vi "LabViewV1.4.0.vi"() -> ()   [LabVIEW 2020]
uses:
  <vilib>/DAQmx/read.llb/DAQmx Read (Analog 2D DBL NChan NSamp).vi
  <vilib>/Analysis/baseanly.llb/Mean (DBL).vi
  <vilib>/DAQmx/miscellaneous.llb/DAQmx Fill In Error Info.vi
  <vilib>/Analysis/NI_AALBase.lvlib
  <resource>/objmgr/daqmx.rc
panel:
  out "Numeric 2":i32
  out "Numeric":i32
  out "index of Module 3":i32
  out "index of Module 2":i32
  out "double precision float":dbl
  out "Time Stamp":timestamp=timestamp(-21600 s since 1904-01-01)
  out "subarray 2":string[](array[string])
  out "index of Module 1":i32
  out "subarray":string[](array[string])
  in  "Counter":dbl
  out ".not. (x .or. y)?":bool
  out "index of element":i32
  out "element":dbl
  out "?":timestamp
  out "Channels":refnum<k21>[](array[refnum])
  out "size(s)":i32
  out "NumDevices":u32
  out "x/y":dbl
  in  "?":T1(tab)
  out "Sampling Status":bool
  in  "Sampling Time":u32=5
  in  "Read Time (s)":u32=60
  in  "Channel List":string(combo)="Temperature"
  out "Read Count Daily":string="0" caption="Timestamp"
  out "Countdown to Read":string="0\n 6:17:48 PM" caption="Timestamp"
  out "?":string="Timestamp"
  out "?":string="File Location"
  out "Timestamp":string="7/26/2020\n 6:17:48 PM"
  in  "Start":bool
  in  "Next Button":bool
  in  "Stop Button 2":bool
  out "Graph Running":bool
  in  "Resolution":u8=10 min=10
  in  "Stop Button":bool
  in  "Play Button":bool
  out "Module 3":bool
  out "Module 2":bool
  out "Module 1":bool
  out "3":bool
  out "2":bool
  out "1":bool
  in  "Running Module":u8=1 min=1 max=3
  in  "Module 3 Task":refnum<k21>="MyTemperatureTask_2"
  out "?":waveform(dbl)(graph)
  in  "Module 3 File Data Location":path=path "E:/KMUTT/Master Degree/labviewjgsee/log/Module3"
  in  "Module 2 File Data Location":path=path "E:/KMUTT/Master Degree/labviewjgsee/log/Module2"
  in  "Module 2 Task":refnum<k21>="MyTemperatureTask_1"
  in  "Module 1 File Data Location":path=path "E:/KMUTT/Master Degree/labviewjgsee/log/Module1"
  in  "Module 1 Task":refnum<k21>="MyTemperatureTask"
  in  "DAQmx Device Name":tag="JGSEE"
  out "Tnp_in":dbl format="%#_4g"
  out "T_head":dbl format="%#_4g"
  out "Tnw":dbl format="%#_4g"
  out "Trp_out":dbl format="%#_4g"
  out "Trp_in":dbl format="%#_4g"
  out "Tww_o":dbl format="%#_4g"
  out "Tew_o":dbl format="%#_4g"
  out "Tsw_o":dbl format="%#_4g"
  out "Tnw_o":dbl format="%#_4g"
  out "3_inlet_HE":dbl format="%#_4g"
  out "tnp_out":dbl format="%#_4g"
  out "4_outlet_HE":dbl format="%#_4g"
  out "Tp5":dbl format="%#_4g"
  out "Tp4":dbl format="%#_4g"
  out "Tp3":dbl format="%#_4g"
  out "Tp2":dbl format="%#_4g"
  out "Tp1":dbl format="%#_4g"
  out "Tnp_o":dbl format="%#_4g"
  out "Tfoot":dbl format="%#_4g"
  out "Ttest":dbl format="%#_4g"
  out "T_body":dbl format="%#_4g"
  out "Tshaft_supply":dbl format="%#_4g"
  out "Tshaft_return":dbl format="%#_4g"
  out "Tat":dbl format="%#_4g"
  out "Ta":dbl format="%#_4g"
  out "Tc":dbl format="%#_4g"
  out "Tf":dbl format="%#_4g"
  out "Tsg":dbl format="%#_4g"
  out "Tew":dbl format="%#_4g"
  out "Tng":dbl format="%#_4g"
  out "Tww":dbl format="%#_4g"
  out "Tsw":dbl format="%#_4g"
  out "Table Module 1":string[][](table)
  out "Table Module 2":string[][](table)
  out "Table Module 3":string[][](table)
  in  "Select Channel Module 1":string(combo)
  out "?":string="Date"
  out "Timestamp 2":string="7/26/2020\n 6:17:48 PM" caption="Timestamp"
  out "Graph Module 1":cluster{timestamp[], dbl[]}[](graph)
  in  "Select Channel Module 2":string(combo)
  out "?":string="Date"
  out "Timestamp 3":string="7/26/2020\n 6:17:48 PM" caption="Timestamp"
  out "Graph Module 2":cluster{timestamp[], dbl[]}[](graph)
  in  "Select Channel Module 3":string(combo)
  out "?":string="Date"
  out "Timestamp 4":string="7/26/2020\n 6:17:48 PM" caption="Timestamp"
  out "Graph Module 3":cluster{timestamp[], dbl[]}[](graph)
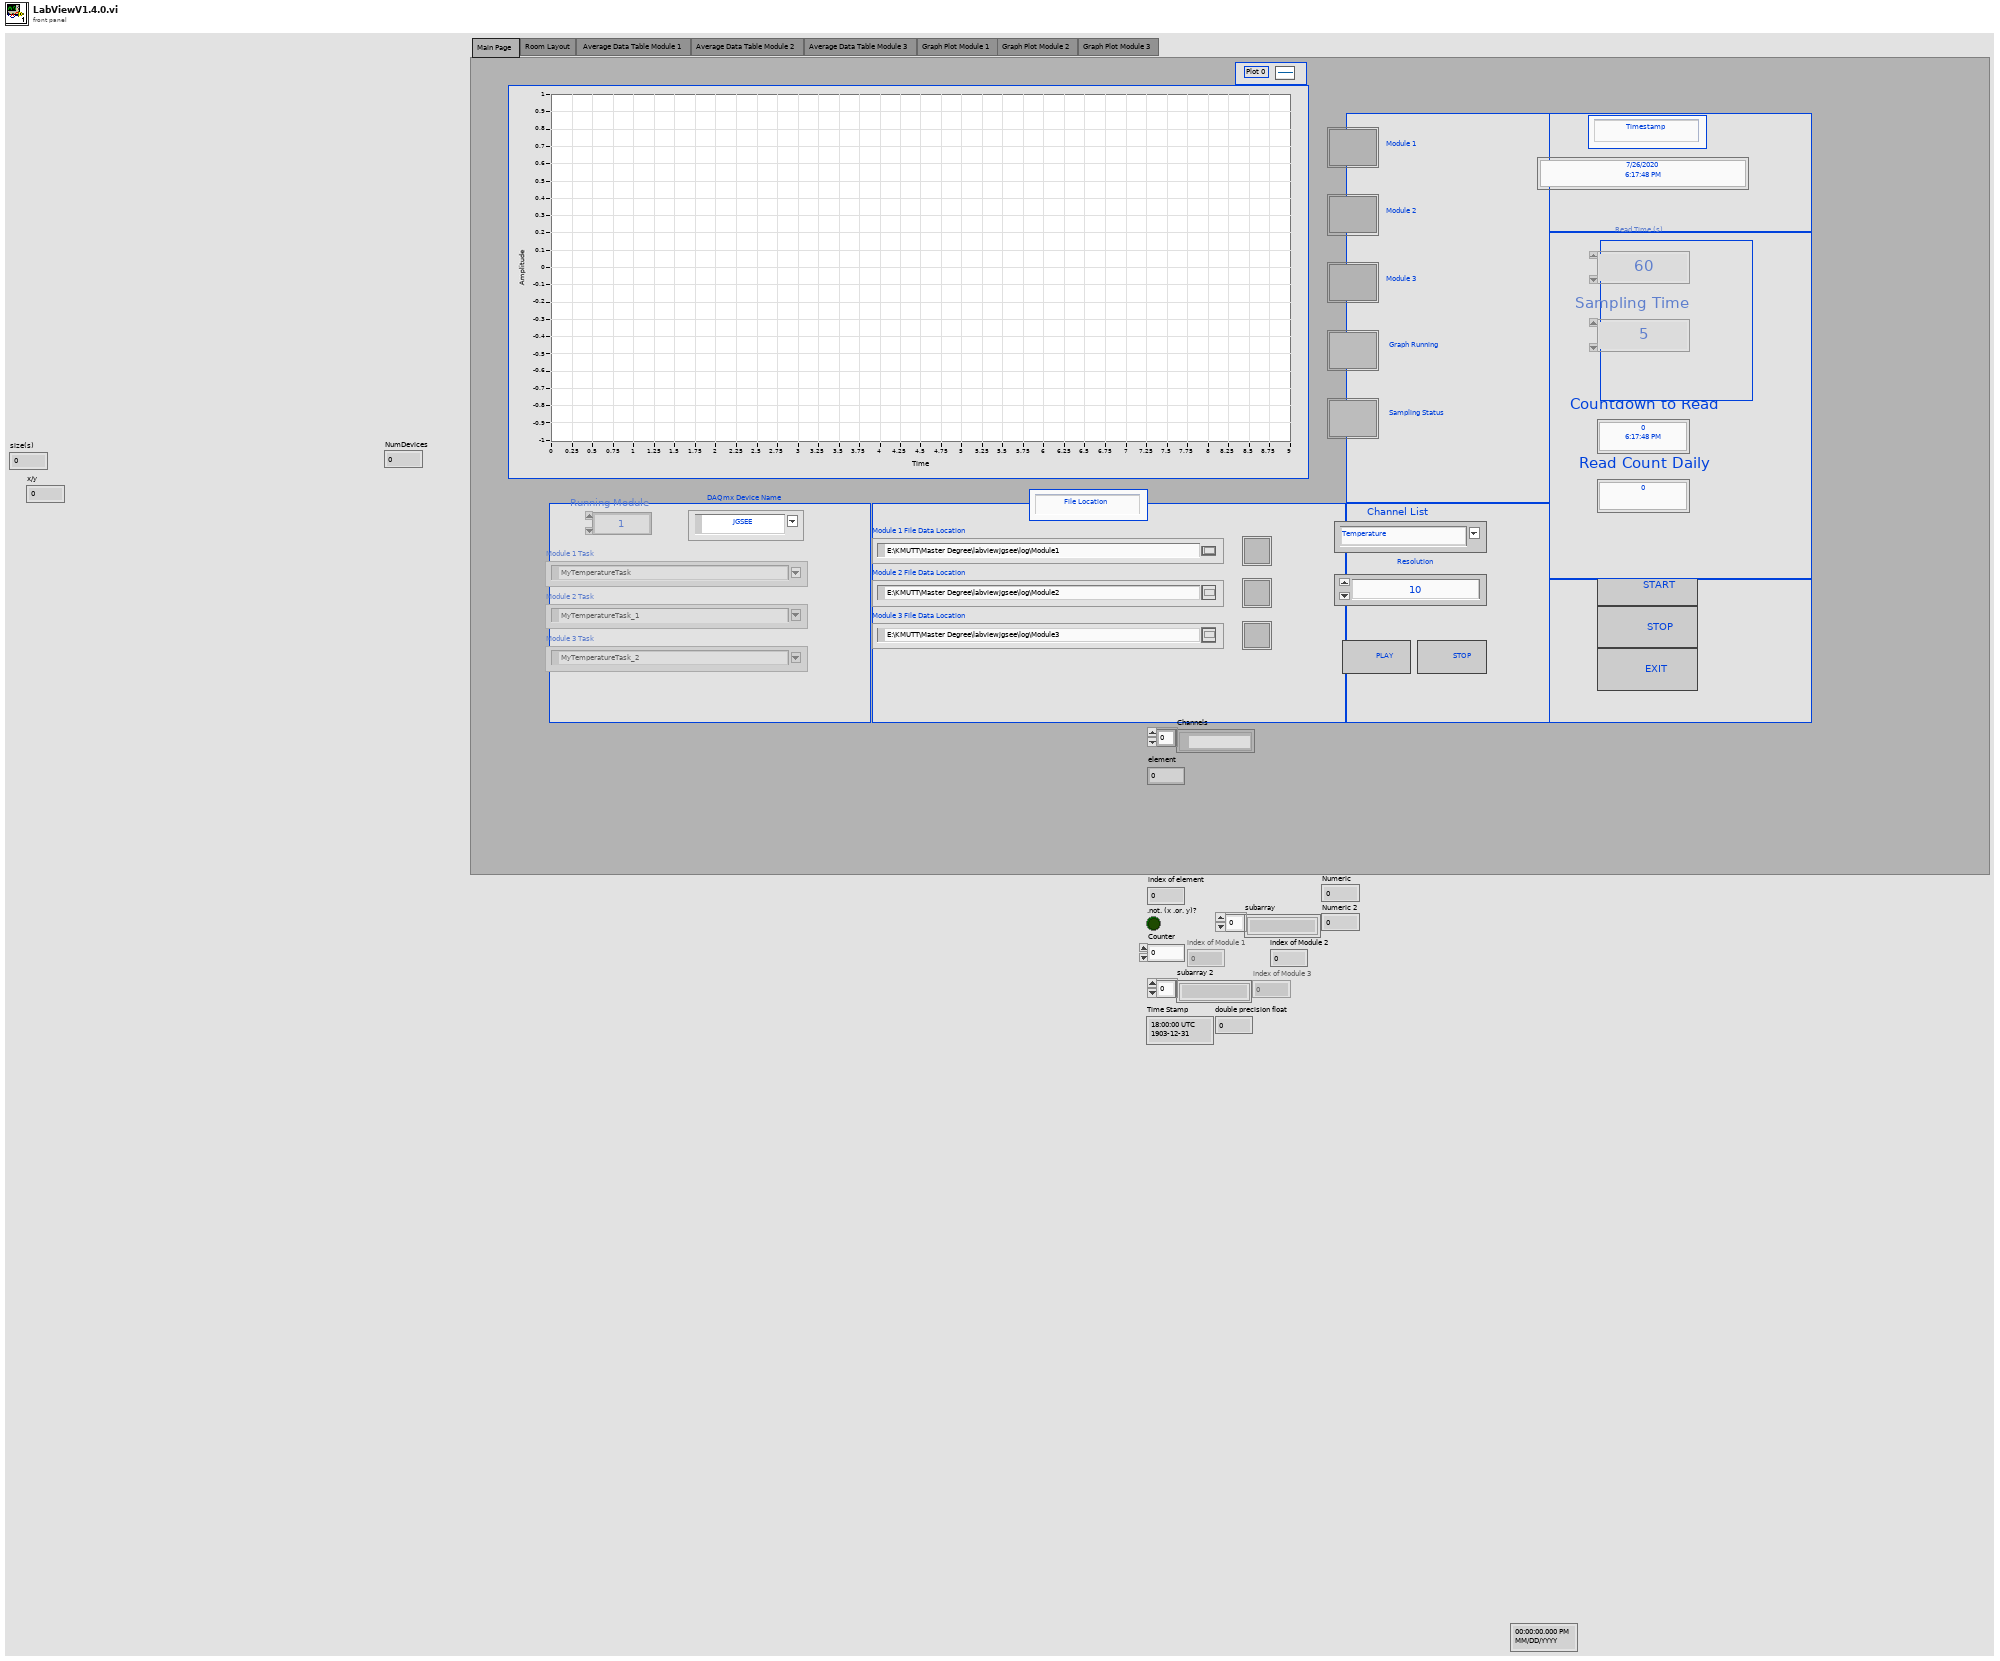
[diagram p1: front panel]
types:
  T1 = enum32{"Main Page ", "Room Layout", " Average Data Table Module 1", "Average Data Table Module 2", "Average Data Table Module 3", "Graph Plot Module 1", "Graph Plot Module 2", "Graph Plot Module 3"}
  T2 = enum16{"open", "replace", "create", "open or create", "replace or create", "replace or create with confirmation"}
  T3 = enum8{"Enabled", "Disabled", "Disabled and Grayed Out"}
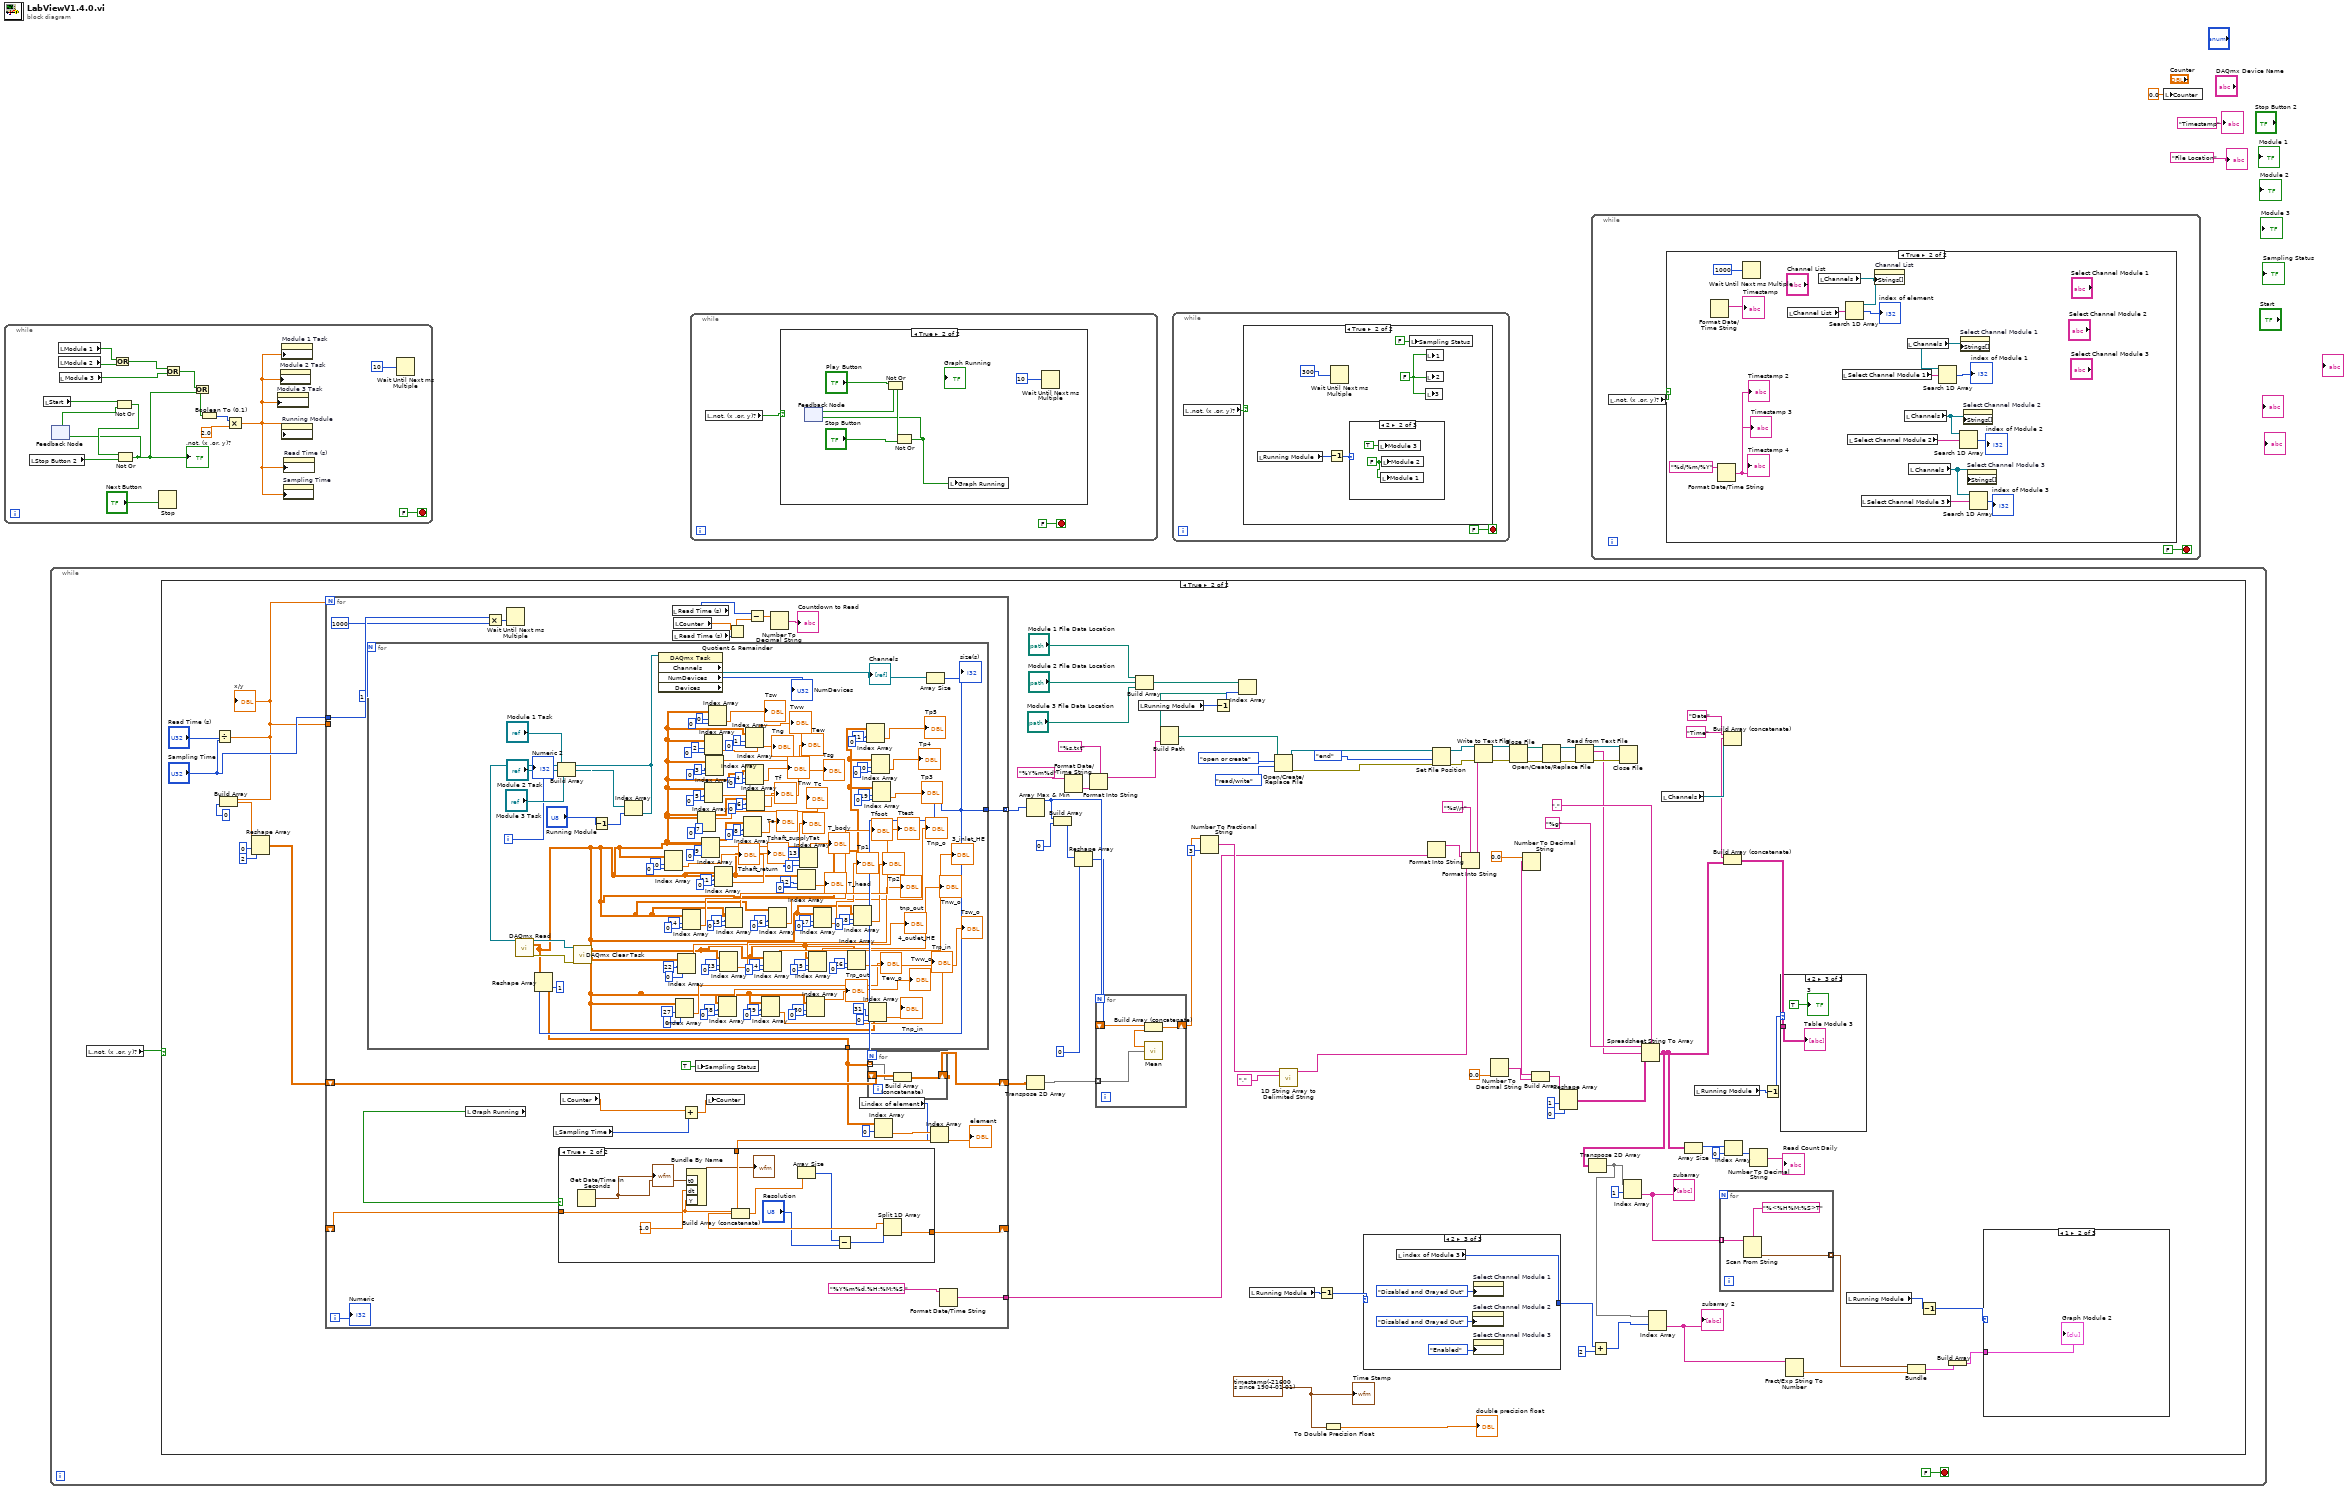
[diagram p0: block diagram]
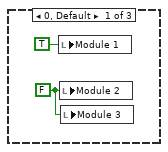
[diagram p4: hidden frame]
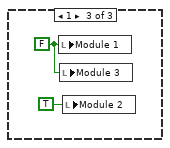
[diagram p5: hidden frame]
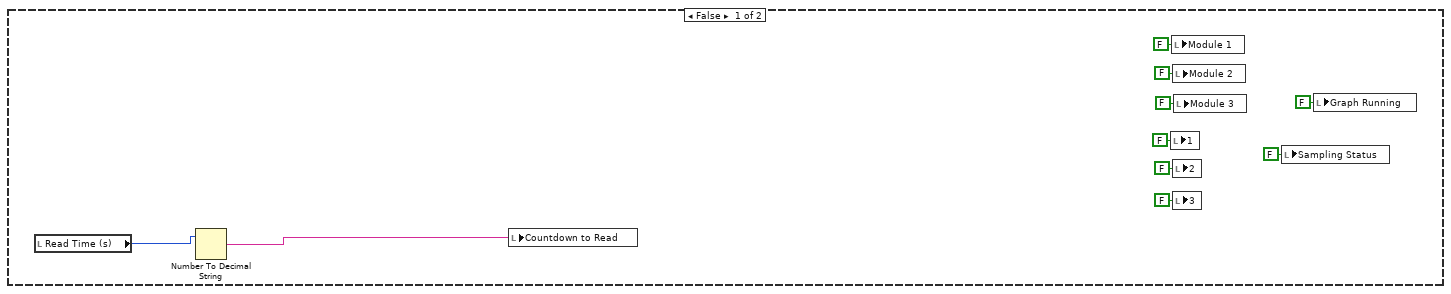
[diagram p7: hidden frame]
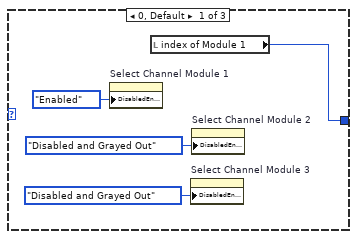
[diagram p8: hidden frame]
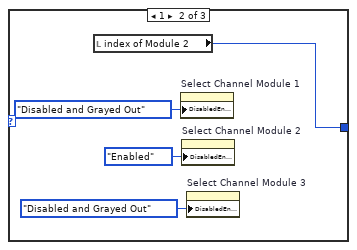
[diagram p9: hidden frame]
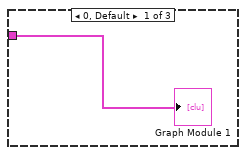
[diagram p10: hidden frame]
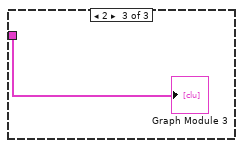
[diagram p11: hidden frame]
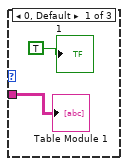
[diagram p12: hidden frame]
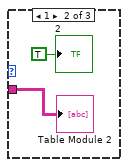
[diagram p13: hidden frame]
diagram:
  n1 = while {
    stop <- FALSE stop-if-true
    n2 = local read "Stop Button 2"() -> (w19:bool)
    n3 = local read "Start"() -> (w15:bool)
    n4 = feedback #1() -> (w17:bool)  [unwired: 1 in]
    n5 = local read "Module 1"() -> (w13:bool)
    n6 = local read "Module 2"() -> (w12:bool)
    n7 = local read "Module 3"() -> (w10:bool)
    n8 = Or(x=w13, y=w12) -> (x .or. y?=w11:bool)
    n9 = Not Or(1:w17, 2:w15) -> (0:w18:bool)
    n10 = Not Or(1:w19, 2:w18) -> (0:w7:bool)
    ".not. (x .or. y)?" <- w7
    n11 = feedback-in #1(w7) -> ()
    n12 = Stop(stop? (T)="Next Button") -> ()
    n13 = Or(x=w11, y=w10) -> (x .or. y?=w9:bool)
    n14 = Or(x=w9, y=w7) -> (x .or. y?=w6:bool)
    n15 = Boolean To (0,1)(Boolean=w6) -> (0, 1=w8:i16)
    n16 = Multiply(x=w8, y=2.0) -> (x*y=w5:dbl)
    n17 = property on="Module 3 Task" class="DAQmxName (strict)"("DisabledEnum"=w5) -> ()  [unwired: 2 in, 2 out]
    n18 = property on="Module 2 Task" class="DAQmxName (strict)"("DisabledEnum"=w5) -> ()  [unwired: 2 in, 2 out]
    n19 = property on="Module 1 Task" class="DAQmxName (strict)"("DisabledEnum"=w5) -> ()  [unwired: 2 in, 2 out]
    n20 = property on="Running Module" class="DigNum (strict)"("DisabledEnum"=w5) -> ()  [unwired: 2 in, 2 out]
    n21 = property on="Sampling Time" class="DigNum (strict)"("DisabledEnum"=w5) -> ()  [unwired: 2 in, 2 out]
    n22 = property on="Read Time (s)" class="DigNum (strict)"("DisabledEnum"=w5) -> ()  [unwired: 2 in, 2 out]
    n23 = Wait Until Next ms Multiple(millisecond multiple=u32 10 ("milliseconds to wait")) -> ()  [unwired: 1 out]
  }
  n24 = while {
    stop <- FALSE stop-if-true
    n25 = local read ".not. (x .or. y)?"() -> (w21:bool)
    n26 = case shown="True" w21 {
      frame False {
        n27 = local read "Read Time (s)"() -> (w24:u32)
        n28 = Number To Decimal String(number=w24) -> (decimal integer string=w23:string)  [unwired: 1 in]
        n29 = local write "Countdown to Read"(w23) -> ()
        n30 = local write "1"(FALSE ("1")) -> ()
        n31 = local write "Module 1"(FALSE ("Module 1")) -> ()
        n32 = local write "Module 2"(FALSE ("Module 2")) -> ()
        n33 = local write "2"(FALSE ("2")) -> ()
        n34 = local write "3"(FALSE ("3")) -> ()
        n35 = local write "Module 3"(FALSE ("Module 3")) -> ()
        n36 = local write "Sampling Status"(FALSE ("Sampling Status")) -> ()
        n37 = local write "Graph Running"(FALSE ("Graph Running")) -> ()
      }
      frame True {
        w42 = timestamp(-21600 s since 1904-01-01)
        n38 = Divide(x="Read Time (s)", y="Sampling Time") -> (x/y=w34:dbl)
        "x/y" <- w34
        n39 = Build Array(w34, 0 ("element")) -> (w107:dbl[])
        n40 = Reshape Array(w107, 0 ("dimension size"), 2 ("dimension size")) -> (w104:dbl[][])
        n41 = for {
          N: w34 -> [_]
          shift-right: [w176] -> w73
          shift-left: w104 -> [w175]
          tunnel: "Sampling Time" -> [w174]
          tunnel: [w172] -> w103 mode=indexing
          shift-right: [w167] -> _
          shift-left: _ -> [w166]
          tunnel: w34 -> [_]
          tunnel: [w153] -> w33
          i -> [w151]
          n42 = for {
            N: 1 -> [_]
            tunnel: [w286] -> w172
            tunnel: [w274] -> w171
            i -> [w276]
            n43 = Build Array("Module 1 Task", "Module 2 Task", "Module 3 Task") -> (w282:refnum<k21>[])
            n44 = Decrement(x="Running Module") -> (x-1=w278:u8)
            n45 = Index Array(array=w282, index=w278) -> (element=w281:refnum<k21>)
            n46 = call-poly <vilib>:"DAQmx Read.vi"("task/channels in"=w281) -> ("task out"=w287:refnum<k21>, "data"=w180:dbl[][], "error out"=w288:errorcluster)  [unwired: 12 in]
            n47 = call <vilib>:"DAQmx Clear Task.vi"("task in"=w287, "error in"=w288) -> ()  [unwired: 13 in, 1 out]
            n48 = property class="DAQmx Task" props=["Channels", "NumDevices", "Devices"](reference=w281) -> ("Channels"=w277:refnum<k21>[], "NumDevices"=→"NumDevices":u32)  [unwired: 1 in, 3 out]
            "Channels" <- w277
            n49 = Index Array(array=w180, index (row)=10, index (col)=0 ("disabled index (col)")) -> (element=→"Tshaft_return":dbl)
            n50 = Index Array(array=w180, index (row)=27, index (col)=0) -> (element=→"Tew_o":dbl)
            n51 = Index Array(array=w180, index (row)=22, index (col)=0) -> (element=→"4_outlet_HE":dbl)
            n52 = Index Array(array=w180, index (row)=14, index (col)=0 ("disabled index (col)")) -> (element=→"Tfoot":dbl)
            n53 = Index Array(array=w180, index (row)=7, index (col)=0 ("disabled index (col)")) -> (element=→"Tc":dbl)
            n54 = Index Array(array=w180, index (row)=9, index (col)=0 ("disabled index (col)")) -> (element=→"Tat":dbl)
            n55 = Index Array(array=w180, index (row)=2, index (col)=0 ("disabled index (col)")) -> (element=→"Tng":dbl)
            n56 = Index Array(array=w180, index (row)=5, index (col)=0 ("disabled index (col)")) -> (element=→"Tsg":dbl)
            n57 = Index Array(array=w180, index (row)=3, index (col)=0 ("disabled index (col)")) -> (element=→"Tew":dbl)
            n58 = Index Array(array=w180, index (row)=0, index (col)=0 ("disabled index (col)")) -> (element=→"Tsw":dbl)
            n59 = Index Array(array=w180, index (row)=11, index (col)=0 ("disabled index (col)")) -> (element=→"Tshaft_supply":dbl)
            n60 = Index Array(array=w180, index (row)=28, index (col)=0 ("disabled index (col)")) -> (element=→"Tww_o":dbl)
            n61 = Index Array(array=w180, index (row)=23, index (col)=0 ("disabled index (col)")) -> (element=→"tnp_out":dbl)
            n62 = Index Array(array=w180, index (row)=15, index (col)=0 ("disabled index (col)")) -> (element=→"Ttest":dbl)
            n63 = Index Array(array=w180, index (row)=8, index (col)=0 ("disabled index (col)")) -> (element=→"Ta":dbl)
            n64 = Index Array(array=w180, index (row)=1, index (col)=0 ("disabled index (col)")) -> (element=→"Tww":dbl)
            n65 = Index Array(array=w180, index (row)=4, index (col)=0 ("disabled index (col)")) -> (element=→"Tnw":dbl)
            n66 = Index Array(array=w180, index (row)=6, index (col)=0 ("disabled index (col)")) -> (element=→"Tf":dbl)
            n67 = Index Array(array=w180, index (row)=29, index (col)=0 ("disabled index (col)")) -> (element=→"Trp_in":dbl)
            n68 = Index Array(array=w180, index (row)=24, index (col)=0 ("disabled index (col)")) -> (element=→"3_inlet_HE":dbl)
            n69 = Index Array(array=w180, index (row)=16, index (col)=0 ("disabled index (col)")) -> (element=→"Tnp_o":dbl)
            n70 = Index Array(array=w180, index (row)=12, index (col)=0) -> (element=→"T_head":dbl)
            n71 = Index Array(array=w180, index (row)=13, index (col)=0 ("disabled index (col)")) -> (element=→"T_body":dbl)
            n72 = Index Array(array=w180, index (row)=30, index (col)=0 ("disabled index (col)")) -> (element=→"Trp_out":dbl)
            n73 = Index Array(array=w180, index (row)=25, index (col)=0 ("disabled index (col)")) -> (element=→"Tnw_o":dbl)
            n74 = Index Array(array=w180, index (row)=17, index (col)=0 ("disabled index (col)")) -> (element=→"Tp1":dbl)
            n75 = Index Array(array=w180, index (row)=26, index (col)=0 ("disabled index (col)")) -> (element=→"Tsw_o":dbl)
            n76 = Index Array(array=w180, index (row)=18, index (col)=0 ("disabled index (col)")) -> (element=→"Tp2":dbl)
            n77 = Index Array(array=w180, index (row)=21, index (col)=0 ("disabled index (col)")) -> (element=→"Tp5":dbl)
            n78 = Index Array(array=w180, index (row)=31, index (col)=0 ("disabled index (col)")) -> (element=→"Tnp_in":dbl)
            n79 = Index Array(array=w180, index (row)=20, index (col)=0 ("disabled index (col)")) -> (element=→"Tp4":dbl)
            n80 = Index Array(array=w180, index (row)=19, index (col)=0 ("disabled index (col)")) -> (element=→"Tp3":dbl)
            n81 = Array Size(array=w277) -> (size(s)=w286:i32)
            "size(s)" <- w286
            n82 = Reshape Array(w180, 1 ("dimension size"), w286) -> (w274:dbl[][])
            "Numeric 2" <- w276
          }
          n83 = local read "Graph Running"() -> (w165:bool)
          n84 = Multiply(x=w174, y=u32 1000) -> (x*y=w149:u32)
          n85 = Wait Until Next ms Multiple(millisecond multiple=w149) -> ()  [unwired: 1 out]
          n86 = local read "Sampling Time"() -> (w161:u32)
          n87 = local read "Counter"() -> (w160:dbl)
          n88 = local read "Read Time (s)"() -> (w157:u32)
          n89 = local read "Read Time (s)"() -> (w159:u32)
          n90 = local read "Counter"() -> (w154:dbl)
          n91 = Add(x=w160, y=w161) -> (x+y=w162:dbl)
          n92 = local write "Sampling Status"(TRUE ("Sampling Status")) -> ()
          n93 = local write "Counter"(w162) -> ()
          n94 = Quotient & Remainder(x=w154, y=w159) -> (x-y*floor(x/y)=w158:dbl)  [unwired: 1 out]
          n95 = Subtract(x=w157, y=w158) -> (x-y=w156:dbl)
          n96 = Number To Decimal String(number=w156) -> (decimal integer string=→"Countdown to Read":string)  [unwired: 1 in]
          n97 = local read "index of element"() -> (w164:i32)
          n98 = for {
            N: w172 -> [_]
            shift-right: [w300] -> w176
            shift-left: w175 -> [w301]
            tunnel: w171 -> [w299] mode=indexing
            n99 = Build Array (concatenate)(w301, w299) -> (w300:dbl[][])
          }
          n100 = Index Array(array=w171, index (row)=0) -> (element=w169:dbl[])  [unwired: 1 in]
          n101 = Index Array(array=w169, index=w164) -> (element=w168:dbl)
          "element" <- w168
          n102 = case shown="True" w165 {
            tunnel: w168 -> [_ w296]
            tunnel: [_ w293] -> w167
            tunnel: w166 -> [_ w292]
            frame False {
            }
            frame True {
              n103 = Get Date/Time In Seconds() -> (seconds since 1Jan1904=w298:timestamp)
              "?" <- w298
              n104 = Bundle By Name("t0"=w298, "dt"=1.0, "Y"=w292) -> (→"?":waveform(dbl))  [unwired: 1 in]
              n105 = Build Array (concatenate)(w292, w296) -> (w294:dbl[])
              n106 = Array Size(array=w294) -> (size(s)=w290:i32)
              n107 = Subtract(x=w290, y="Resolution") -> (x-y=w291:i32)
              n108 = Split 1D Array(array=w294, index=w291) -> (second subarray=w293:dbl[])  [unwired: 1 out]
            }
          }
          n109 = Format Date/Time String(time format string (%c)="%Y%m%d,%H:%M:%S,") -> (date/time string=w153:string)  [unwired: 2 in]
          "Numeric" <- w151
        }
        n110 = Array Max & Min(array=w103) -> (max value=w100:i32)  [unwired: 3 out]
        n111 = Transpose 2D Array(2D array=w73) -> (transposed array=w102:dbl[][])
        n112 = Build Array(w100, 0 ("element")) -> (w98:i32[])
        n113 = Format Date/Time String(time format string (%c)="%Y%m%d") -> (date/time string=w117:string)  [unwired: 2 in]
        n114 = Reshape Array(w98, 0 ("dimension size")) -> (w97:i32[])
        n115 = Format Into String(format string="%s.txt", w117) -> (resulting string=w115:string)  [unwired: 2 in, 1 out]
        n116 = for {
          N: w100 -> [_]
          tunnel: w102 -> [w305] mode=indexing
          shift-right: [w303] -> w109
          shift-left: w97 -> [w302]
          n117 = call-poly <vilib>:"Mean.vi"("X"=w305) -> ("mean"=w304:dbl)  [unwired: 1 out]
          n118 = Build Array (concatenate)(w302, w304) -> (w303:dbl[])
        }
        n119 = Build Array("Module 1 File Data Location", "Module 2 File Data Location", "Module 3 File Data Location") -> (w66:path[])
        n120 = local read "Running Module"() -> (w67:u8)
        n121 = Number To Fractional String(number=w109, precision (6)=i16 3) -> (F-format string=w110:string[])  [unwired: 2 in]
        n122 = Decrement(x=w67) -> (x-1=w65:u8)
        n123 = Index Array(array=w66, index=w65) -> (element=w64:path)
        n124 = Build Path(base path=w64, name or relative path=w115) -> (appended path=w114:path)
        n125 = local read "Running Module"() -> (w40:u8)
        n126 = Open/Create/Replace File(file path (use dialog)=w114, operation (0:open)=T2."open or create", access (0:read/write)=enum16{"read/write", "read-only", "write-only"}."read/write") -> (refnum out=w95:refnum<file>, error out=w121:errorcluster)  [unwired: 3 in, 1 out]
        n127 = call <vilib>:"1D String Array to Delimited String.vi"("delimiter"="," ("format string"), "string array"=w110) -> ("delimited string"=w113:string)  [unwired: 9 in]
        n128 = Decrement(x=w40) -> (x-1=w39:u8)
        n129 = To Double Precision Float(number=w42) -> (double precision float=→"double precision float":dbl)
        n130 = case shown="2" w39 {
          tunnel: [w128 w132 w136] -> w35
          frame 0, Default {
            n131 = property on="Select Channel Module 1" class="CmbBox"("DisabledEnum"=T3."Enabled" ("Disabled")) -> ()  [unwired: 2 in, 2 out]
            n132 = local read "index of Module 1"() -> (w128:i32)
            n133 = property on="Select Channel Module 3" class="CmbBox"("DisabledEnum"=T3."Disabled and Grayed Out" ("Disabled")) -> ()  [unwired: 2 in, 2 out]
            n134 = property on="Select Channel Module 2" class="CmbBox"("DisabledEnum"=T3."Disabled and Grayed Out" ("Disabled")) -> ()  [unwired: 2 in, 2 out]
          }
          frame 1 {
            n135 = local read "index of Module 2"() -> (w132:i32)
            n136 = property on="Select Channel Module 1" class="CmbBox"("DisabledEnum"=T3."Disabled and Grayed Out" ("Disabled")) -> ()  [unwired: 2 in, 2 out]
            n137 = property on="Select Channel Module 2" class="CmbBox"("DisabledEnum"=T3."Enabled" ("Disabled")) -> ()  [unwired: 2 in, 2 out]
            n138 = property on="Select Channel Module 3" class="CmbBox"("DisabledEnum"=T3."Disabled and Grayed Out" ("Disabled")) -> ()  [unwired: 2 in, 2 out]
          }
          frame 2 {
            n139 = local read "index of Module 3"() -> (w136:i32)
            n140 = property on="Select Channel Module 2" class="CmbBox"("DisabledEnum"=T3."Disabled and Grayed Out" ("Disabled")) -> ()  [unwired: 2 in, 2 out]
            n141 = property on="Select Channel Module 1" class="CmbBox"("DisabledEnum"=T3."Disabled and Grayed Out" ("Disabled")) -> ()  [unwired: 2 in, 2 out]
            n142 = property on="Select Channel Module 3" class="CmbBox"("DisabledEnum"=T3."Enabled" ("Disabled")) -> ()  [unwired: 2 in, 2 out]
          }
        }
        n143 = Format Into String(w33) -> (resulting string=w111:string)  [unwired: 3 in, 1 out]
        n144 = Set File Position(refnum=w95, from (0:start)=enum16{"start", "end", "current"}."end", error in=w121) -> (refnum out=w122:refnum<file>, error out=w120:errorcluster)  [unwired: 1 in]
        n145 = Format Into String(format string="%s\\n", initial string=w111, w113) -> (resulting string=w87:string)  [unwired: 1 in, 1 out]
        n146 = Write to Text File(file (use dialog)=w122, text=w87, error in=w120) -> (refnum out=w94:refnum<file>, error out=w93:errorcluster)  [unwired: 1 in, 1 out]
        n147 = Number To Decimal String(number=0.0 ("element")) -> (decimal integer string=w75:string)  [unwired: 1 in]
        n148 = Close File(refnum=w94, error in=w93) -> (path=w92:path, error out=w91:errorcluster)
        n149 = Number To Decimal String(number=0.0 ("element")) -> (decimal integer string=w77:string)  [unwired: 1 in]
        n150 = Build Array(w77, w75) -> (w79:string[])
        n151 = Open/Create/Replace File(file path (use dialog)=w92, error in=w91) -> (refnum out=w90:refnum<file>, error out=w89:errorcluster)  [unwired: 4 in, 1 out]
        n152 = Reshape Array(w79, 1 ("dimension size"), 0 ("dimension size")) -> (w80:string[][])
        n153 = Read from Text File(file (use dialog)=w90, error in=w89) -> (refnum out=w88:refnum<file>, text=w83:string, error out=w84:errorcluster)  [unwired: 2 in, 1 out]
        n154 = Add(x=w35, y=2) -> (x+y=w48:i32)
        n155 = Close File(refnum=w88, error in=w84) -> ()  [unwired: 2 out]
        n156 = Spreadsheet String To Array(delimiter (Tab)=",", format string="%g", spreadsheet string=w83, array type (2D Dbl)=w80) -> (array=w52:string[][])
        n157 = Transpose 2D Array(2D array=w52) -> (transposed array=w49:string[][])
        n158 = Index Array(array=w49, index (row)=1 ("index")) -> (element=w47:string[])  [unwired: 1 in]
        "subarray" <- w47
        n159 = Index Array(array=w49, index (row)=w48) -> (element=w45:string[])  [unwired: 1 in]
        "subarray 2" <- w45
        n160 = local read "Channels"() -> (w58:refnum<k21>[])
        n161 = Array Size(array=w52) -> (size(s)=w56:i32[])
        n162 = local read "Running Module"() -> (w63:u8)
        n163 = for {
          tunnel: w47 -> [w141] mode=indexing
          tunnel: [w140] -> w43 mode=indexing
          n164 = Scan From String(format string="%<%H%M:%S>T", input string=w141) -> (output 1=w140:timestamp)  [unwired: 3 in, 3 out]
        }
        n165 = Build Array (concatenate)("Date", "Time", w58) -> (w57:string[])
        n166 = Build Array (concatenate)(w57, w52) -> (w61:string[][])
        n167 = Index Array(array=w56, index=0) -> (element=w54:i32)
        n168 = Number To Decimal String(number=w54) -> (decimal integer string=→"Read Count Daily":string)  [unwired: 1 in]
        n169 = Decrement(x=w63) -> (x-1=w62:u8)
        n170 = case shown="2" w62 {
          tunnel: w61 -> [w144 w146 w148]
          frame 0, Default {
            "Table Module 1" <- w144
            "1" <- TRUE ("1")
          }
          frame 1 {
            "Table Module 2" <- w146
            "2" <- TRUE ("2")
          }
          frame 2 {
            "Table Module 3" <- w148
            "3" <- TRUE ("3")
          }
        }
        n171 = Fract/Exp String To Number(string=w45) -> (number=w44:dbl[])  [unwired: 3 in, 1 out]
        n172 = local read "Running Module"() -> (w38:u8)
        n173 = Bundle(w43, w44) -> (w46:cluster{timestamp[], dbl[]})  [unwired: 1 in]
        n174 = Decrement(x=w38) -> (x-1=w37:u8)
        n175 = Build Array(w46) -> (w36:cluster{timestamp[], dbl[]}[])
        n176 = case shown="1" w37 {
          tunnel: w36 -> [w137 w138 w139]
          frame 0, Default {
            "Graph Module 1" <- w137
          }
          frame 1 {
            "Graph Module 2" <- w138
          }
          frame 2 {
            "Graph Module 3" <- w139
          }
        }
        "Time Stamp" <- w42
      }
    }
  }
  n177 = while {
    stop <- FALSE stop-if-true
    n178 = local read ".not. (x .or. y)?"() -> (w306:bool)
    n179 = case shown="True" w306 {
      frame False {
      }
      frame True {
        n180 = feedback #2() -> (w310:bool)  [unwired: 1 in]
        n181 = Not Or(1:w310, 2:"Play Button") -> (0:w311:bool)
        n182 = Not Or(1:"Stop Button", 2:w311) -> (0:w309:bool)
        n183 = feedback-in #2(w309) -> ()
        n184 = local write "Graph Running"(w309) -> ()
        n185 = Wait Until Next ms Multiple(millisecond multiple=u32 10 ("milliseconds to wait")) -> ()  [unwired: 1 out]
      }
    }
  }
  n186 = while {
    stop <- FALSE stop-if-true
    n187 = local read ".not. (x .or. y)?"() -> (w314:bool)
    n188 = case shown="True" w314 {
      frame False {
      }
      frame True {
        w319 = FALSE ("1")
        n189 = local read "Running Module"() -> (w318:u8)
        n190 = Decrement(x=w318) -> (x-1=w317:u8)
        n191 = Wait Until Next ms Multiple(millisecond multiple=u32 300 ("milliseconds to wait")) -> ()  [unwired: 1 out]
        n192 = case shown="2" w317 {
          frame 0, Default {
            w322 = FALSE ("Module 2")
            n193 = local write "Module 1"(TRUE ("Module 1")) -> ()
            n194 = local write "Module 2"(w322) -> ()
            n195 = local write "Module 3"(w322) -> ()
          }
          frame 2 {
            w324 = FALSE ("Module 2")
            n196 = local write "Module 3"(TRUE ("Module 3")) -> ()
            n197 = local write "Module 1"(w324) -> ()
            n198 = local write "Module 2"(w324) -> ()
          }
          frame 1 {
            w326 = FALSE ("Module 1")
            n199 = local write "Module 1"(w326) -> ()
            n200 = local write "Module 3"(w326) -> ()
            n201 = local write "Module 2"(TRUE ("Module 2")) -> ()
          }
        }
        n202 = local write "Sampling Status"(FALSE ("Sampling Status")) -> ()
        n203 = local write "3"(w319) -> ()
        n204 = local write "1"(w319) -> ()
        n205 = local write "2"(w319) -> ()
      }
    }
  }
  n206 = while {
    stop <- FALSE stop-if-true
    n207 = local read ".not. (x .or. y)?"() -> (w327:bool)
    n208 = case shown="True" w327 {
      frame False {
      }
      frame True {
        n209 = Format Date/Time String() -> (date/time string=→"Timestamp":string)  [unwired: 3 in]
        n210 = Format Date/Time String(time format string (%c)="%d/%m/%Y") -> (date/time string=→"Timestamp 2" →"Timestamp 3" →"Timestamp 4":string)  [unwired: 2 in]
        n211 = Wait Until Next ms Multiple(millisecond multiple=u32 1000 ("milliseconds to wait")) -> ()  [unwired: 1 out]
        n212 = local read "Channel List"() -> (w343:string)
        n213 = local read "Channels"() -> (w344:refnum<k21>[])
        n214 = local read "Select Channel Module 1"() -> (w340:string)
        n215 = Search 1D Array(1D array=w344, element=w343) -> (index of element=→"index of element":i32)  [unwired: 1 in]
        n216 = local read "Select Channel Module 2"() -> (w338:string)
        n217 = local read "Select Channel Module 3"() -> (w335:string)
        n218 = property on="Channel List" class="CmbBox"("Strings[]"=w344) -> ()  [unwired: 2 in, 2 out]
        n219 = local read "Channels"() -> (w337:refnum<k21>[])
        n220 = local read "Channels"() -> (w341:refnum<k21>[])
        n221 = local read "Channels"() -> (w334:refnum<k21>[])
        n222 = Search 1D Array(1D array=w341, element=w340) -> (index of element=→"index of Module 1":i32)  [unwired: 1 in]
        n223 = Search 1D Array(1D array=w337, element=w338) -> (index of element=→"index of Module 2":i32)  [unwired: 1 in]
        n224 = property on="Select Channel Module 1" class="CmbBox"("Strings[]"=w341) -> ()  [unwired: 2 in, 2 out]
        n225 = property on="Select Channel Module 2" class="CmbBox"("Strings[]"=w337) -> ()  [unwired: 2 in, 2 out]
        n226 = property on="Select Channel Module 3" class="CmbBox"("Strings[]"=w334) -> ()  [unwired: 2 in, 2 out]
        n227 = Search 1D Array(1D array=w334, element=w335) -> (index of element=→"index of Module 3":i32)  [unwired: 1 in]
      }
    }
  }
  n228 = local write "Counter"(0.0 ("Counter")) -> ()
  "?" <- "File Location" ("String")
  "?" <- "Timestamp"
